vi "Get Configuration Variant Array.vi"(8 "error in":errorcluster, 11 "Master Controller in":refnum<class "EMS User Interface.lvclass">) -> (0 "error out":errorcluster, 2 "Configuration Variant Array":variant[](array[variant]), 3 "Master Controller out":refnum<class "EMS User Interface.lvclass">)   [LabVIEW 2016]
uses:
  EMS Generic.lvclass
  EMS User Interface Actor/EMS User Interface/EMS User Interface.lvclass
  C:/Users/Administrator/Desktop/LabVIEW EMS/EMS Generic Actor/EMS Generic/EMS Generic.lvclass
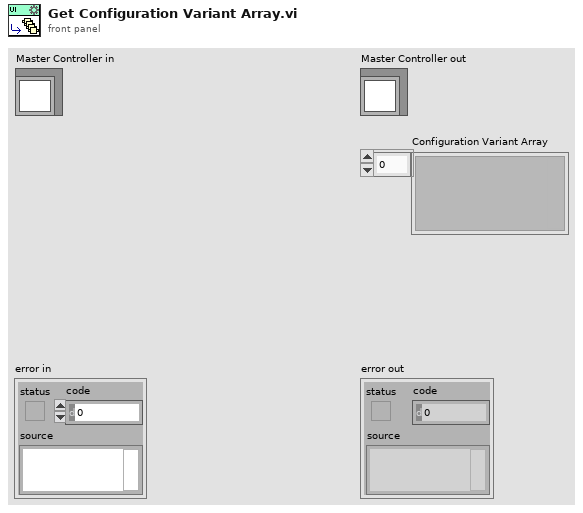
[diagram p1: front panel]
types:
  T1 = typedef "EMS Generic Actor.lvlib/EMS Generic.lvclass/Instance Configuration.ctl" = cluster{"Microgrid ID":u8, "DeviceID":T2, "Device ID Array":T2[], "Nominal Voltage":dbl, "Nominal Frequency":dbl, "Resynch Timeout":i32, "Island Failure Timeout(sec)":dbl}
  T2 = typedef "CSEISMIC DDS.lvlib/CSEISMIC DDS.lvclass/DeviceID.ctl" = string
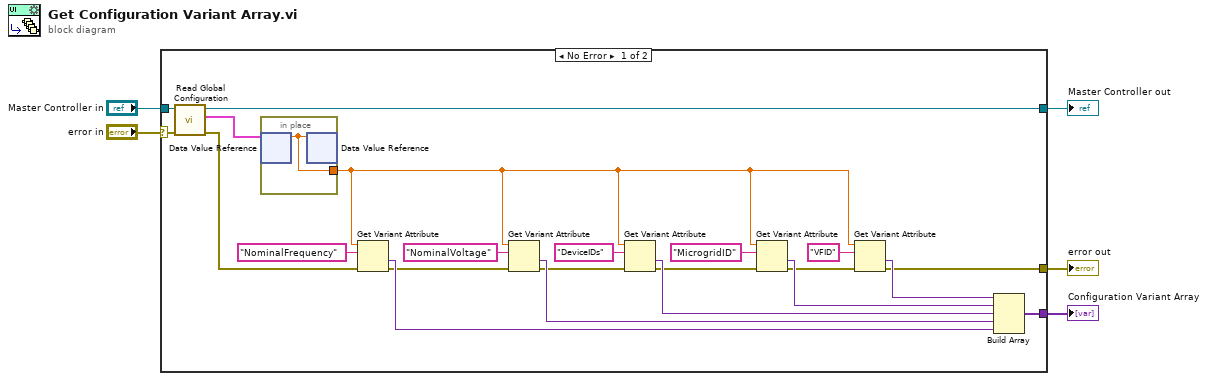
[diagram p0: block diagram]
diagram:
  n1 = case shown="No Error" "error in" {
    selector: "error in" -> [w10 w30]
    tunnel: [w11 w30] -> w4
    tunnel: [w6 w29] -> w2
    tunnel: "Master Controller in" -> [w7 w29]
    tunnel: [w19 _] -> w1
    frame No Error {
      n2 = call "Read Global Configuration.vi"("error in"=w10, "EMS Generic in"=w7) -> ("error out"=w9:errorcluster, "Global Configuration"=w8:T1, "dup EMS Generic out"=w6:refnum<class "EMS User Interface.lvclass">)  [unwired: 7 in]
      n3 = in-place {
        in-place-border: [w28] -> w13
        n4 = in-place-dvr #1(w8) -> (w28:dbl)  [unwired: 1 out]
        n5 = in-place-dvr #1(w28) -> ()  [unwired: 2 out]
      }
      n6 = Get Variant Attribute(Variant=w13, name="NominalFrequency", error in=w9) -> (value=w27:variant, error out=w18:errorcluster)  [unwired: 1 in, 2 out]
      n7 = Get Variant Attribute(Variant=w13, name="NominalVoltage", error in=w18) -> (value=w26:variant, error out=w17:errorcluster)  [unwired: 1 in, 2 out]
      n8 = Get Variant Attribute(Variant=w13, name="DeviceIDs", error in=w17) -> (value=w22:variant, error out=w16:errorcluster)  [unwired: 1 in, 2 out]
      n9 = Get Variant Attribute(Variant=w13, name="MicrogridID", error in=w16) -> (value=w21:variant, error out=w14:errorcluster)  [unwired: 1 in, 2 out]
      n10 = Get Variant Attribute(Variant=w13, name="VFID", error in=w14) -> (value=w12:variant, error out=w11:errorcluster)  [unwired: 1 in, 2 out]
      n11 = Build Array(w12, w21, w22, w26, w27) -> (w19:variant[])
    }
    frame Error {
    }
  }
  "error out" <- w4
  "Master Controller out" <- w2
  "Configuration Variant Array" <- w1
